vi "Temperature Conversion.vi"() -> ()   [LabVIEW 2015]
panel:
  in  "Stop":bool
  out "°F":dbl(slide) scale=0.0..200.0
  in  "°C":dbl(slide) scale=0.0..150.0
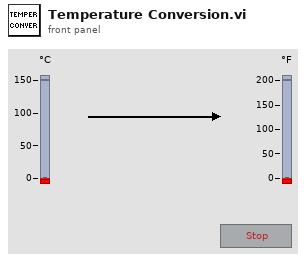
[diagram p1: front panel]
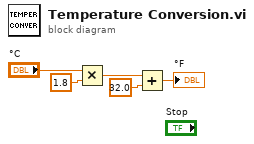
[diagram p0: block diagram]
diagram:
  n1 = Multiply(x="°C", y=1.8) -> (x*y=w3:dbl)
  n2 = Add(x=w3, y=32.0) -> (x+y=→"°F":dbl)
